vi "Initialize.vi"(8 "error in (no error)":errorcluster, 11 "Masterflex Settings in":T1={"VISA resource name"="", "Simulated?"=FALSE, "Pump Number"=1.0, "Reverse?"=FALSE} {"Pump Number" min=1.0 max=20.0 step=1.0}) -> (0 "error out":errorcluster, 1 "Initialized":bool, 2 "No Pump Connected":bool, 3 "Masterflex Settings out":T1={"VISA resource name"="", "Simulated?"=FALSE, "Pump Number"=1.0, "Reverse?"=FALSE} {"Pump Number" min=1.0 max=20.0 step=1.0})   [LabVIEW 2018, in "Masterflex 7550-30.lvlib"]
uses:
  Masterflex 7550-30.lvlib
  Controls/Settings Cluster.ctl
  <vilib>/Instr/_visa.llb/VISA Configure Serial Port (Instr).vi
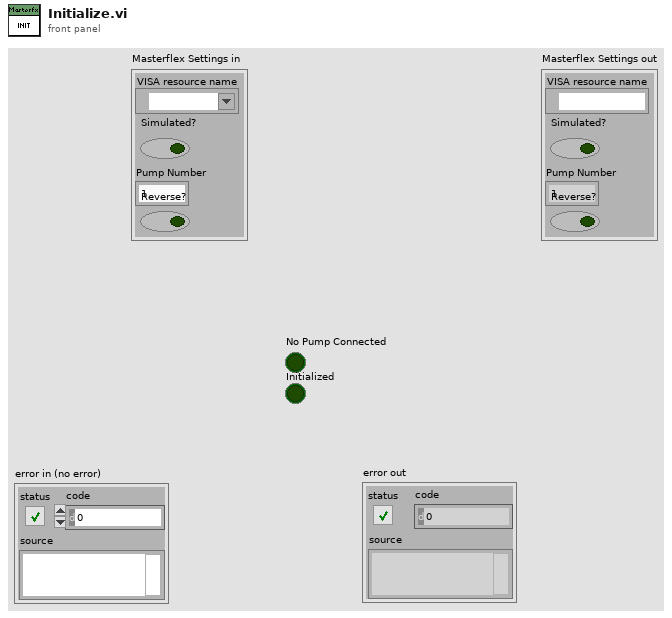
[diagram p1: front panel]
types:
  T1 = typedef "Masterflex 7550-30.lvlib/Settings Cluster.ctl" = cluster{"VISA resource name":refnum<visa-resource-name>, "Simulated?":bool, "Pump Number":dbl, "Reverse?":bool}
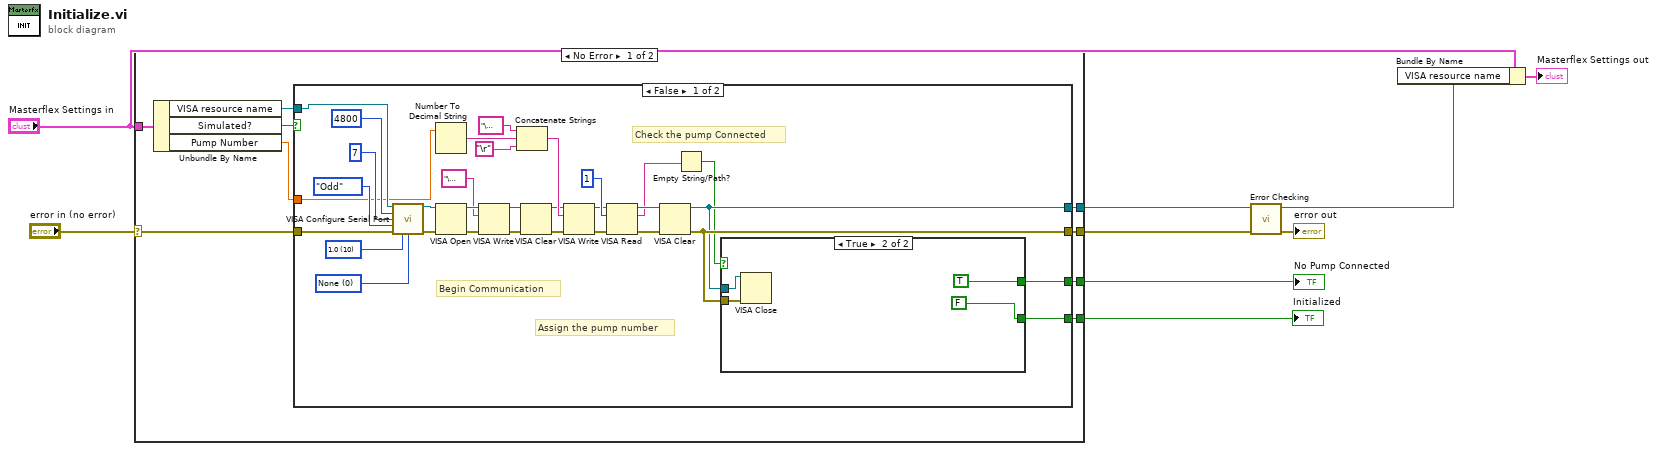
[diagram p0: block diagram]
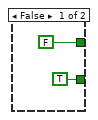
[diagram p2: hidden frame]
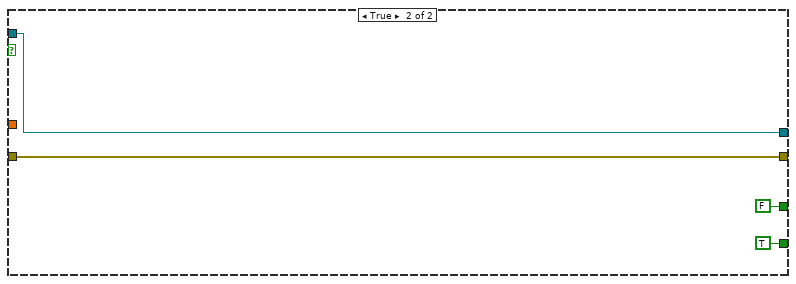
[diagram p3: hidden frame]
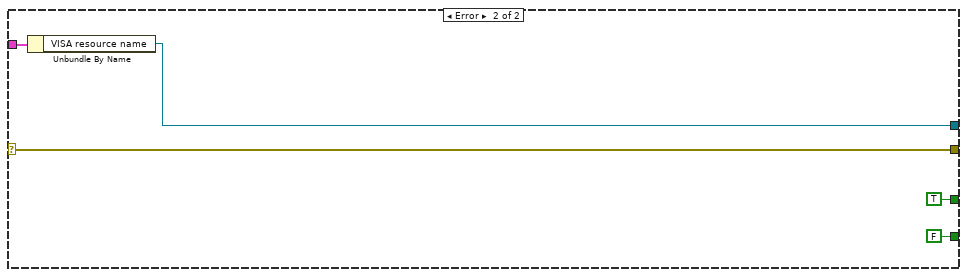
[diagram p4: hidden frame]
diagram:
  n1 = case shown="No Error" "error in (no error)" {
    selector: "error in (no error)" -> [w18 w65]
    tunnel: "Masterflex Settings in" -> [w13 w64]
    tunnel: [w14 w65] -> w6
    tunnel: [w12 w63] -> w3
    tunnel: [w11 FALSE] -> w2
    tunnel: [w10 TRUE] -> w1
    frame No Error {
      n2 = Unbundle By Name(w13) -> ("VISA resource name"=w16:refnum<visa-resource-name>, "Simulated?"=w17:bool, "Pump Number"=w15:dbl)
      n3 = case shown="False" w17 {
        tunnel: w18 -> [w44 w60]
        tunnel: w16 -> [w42 w59]
        tunnel: w15 -> [w34 _]
        tunnel: [w24 w60] -> w14
        tunnel: [w23 w59] -> w12
        tunnel: [w22 TRUE] -> w11
        tunnel: [w21 FALSE] -> w10
        frame False {
          w46 = u16 0 items=["None", "XON/XOFF", "RTS/CTS", "XON/XOFF & RTS/CTS", "DTR/DSR", "XON/XOFF & DTR/DSR"] ("flow control (0:none)")
          w47 = u16 10 items=["1.0"=10, "1.5"=15, "2.0"=20] ("stop bits (10: 1 bit)")
          # "Check the pump Connected"
          # "Assign the pump number"
          # "Begin Communication"
          n4 = call-poly "VISA Configure Serial Port"("VISA resource name"=w42, "baud rate (9600)"=u32 4800, "data bits (8)"=u16 7, "parity (0:none)"=enum16{"None", "Odd", "Even", "Mark", "Space"}."Odd", "error in (no error)"=w44, "stop bits (10: 1 bit)"=w47, "flow control (0:none)"=w46) -> ("VISA resource name out"=w43:refnum<visa-resource-name>, "error out"=w45:errorcluster)  [unwired: 7 in]
          n5 = Number To Decimal String(number=w34) -> (decimal integer string=w35:string)  [unwired: 1 in]
          n6 = VISA Open(error in (no error)=w45, VISA resource name=w43) -> (VISA resource name=w41:refnum<visa-resource-name>, error out=w40:errorcluster)  [unwired: 3 in]
          n7 = VISA Write(VISA resource name=w41, write buffer="\u0005", error in (no error)=w40) -> (VISA resource name out=w30:refnum<visa-resource-name>, error out=w29:errorcluster)  [unwired: 1 out]
          n8 = Concatenate Strings("\u0002" ("string"), w35, "\r") -> (w36:string)
          n9 = VISA Clear(VISA resource name=w30, error in (no error)=w29) -> (VISA resource name out=w28:refnum<visa-resource-name>, error out=w27:errorcluster)
          n10 = VISA Write(VISA resource name=w28, write buffer=w36, error in (no error)=w27) -> (VISA resource name out=w32:refnum<visa-resource-name>, error out=w31:errorcluster)  [unwired: 1 out]
          n11 = VISA Read(VISA resource name=w32, byte count=u32 1, error in (no error)=w31) -> (VISA resource name out=w25:refnum<visa-resource-name>, read buffer=w20:string, error out=w26:errorcluster)  [unwired: 1 out]
          n12 = VISA Clear(VISA resource name=w25, error in (no error)=w26) -> (VISA resource name out=w23:refnum<visa-resource-name>, error out=w24:errorcluster)
          n13 = Empty String/Path?(string/path=w20) -> (empty?=w19:bool)
          n14 = case shown="True" w19 {
            tunnel: w23 -> [_ w56]
            tunnel: w24 -> [_ w55]
            tunnel: [FALSE TRUE] -> w21
            tunnel: [TRUE FALSE] -> w22
            frame False {
            }
            frame True {
              n15 = VISA Close(VISA resource name=w56, error in (no error)=w55) -> ()  [unwired: 1 out]
            }
          }
        }
        frame True {
        }
      }
    }
    frame Error {
      n16 = Unbundle By Name(w64) -> ("VISA resource name"=w63:refnum<visa-resource-name>)
    }
  }
  "Initialized" <- w2
  "No Pump Connected" <- w1
  n17 = call "Error Checking.vi"("error in (no error)"=w6, "VISA resource name"=w3) -> ("error out"=→"error out":errorcluster, "VISA resource name"=w8:refnum<visa-resource-name>)  [unwired: 7 in, 1 out]
  n18 = Bundle By Name(cluster="Masterflex Settings in", "VISA resource name"=w8) -> (→"Masterflex Settings out":T1)
